vi "ColorReader.vi"(1 "file path (dialog if empty)":path=path "C:/Program Files (x86)/FRC Dashboard", 2 "name or relative path":string="Blue.csv") -> (0 "ColorSettings":T1)   [LabVIEW 2013]
uses:
  <vilib>/Utility/file.llb/Read From Spreadsheet File (string).vi
panel:
  out "LumM":i32
  out "Lum":i32
  out "SatM":i32
  out "Sat":i32
  out "HueM":i32
  out "Hue":i32
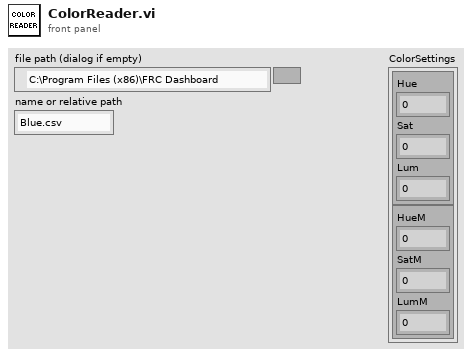
[diagram p1: front panel]
types:
  T1 = cluster{cluster{"Hue":i32, "Sat":i32, "Lum":i32}, cluster{"HueM":i32, "SatM":i32, "LumM":i32}}
  T2 = cluster{"all rows[0]":string, "all rows[1]":string, "all rows[2]":string, "all rows[3]":string, "all rows[4]":string, "all rows[5]":string, "all rows[6]":string, "all rows[7]":string, "all rows[8]":string}
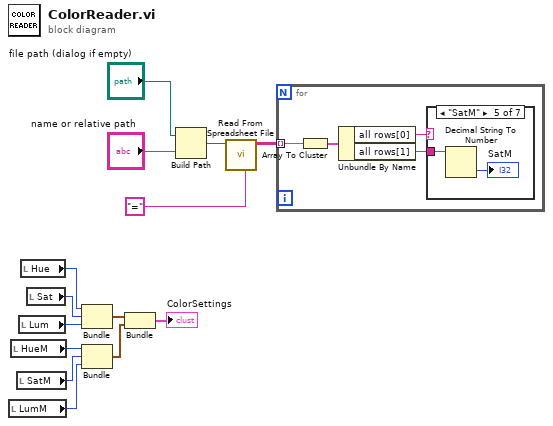
[diagram p0: block diagram]
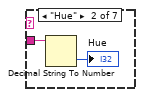
[diagram p3: hidden frame]
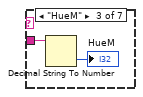
[diagram p4: hidden frame]
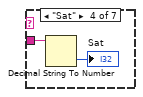
[diagram p5: hidden frame]
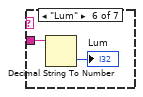
[diagram p6: hidden frame]
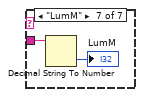
[diagram p7: hidden frame]
diagram:
  n1 = local read "LumM"() -> (w6:i32)
  n2 = local read "HueM"() -> (w9:i32)
  n3 = local read "SatM"() -> (w7:i32)
  n4 = local read "Lum"() -> (w5:i32)
  n5 = local read "Hue"() -> (w8:i32)
  n6 = local read "Sat"() -> (w4:i32)
  n7 = Bundle("Hue"=w8, "Sat"=w4, "Lum"=w5) -> (w10:cluster{"Hue":i32, "Sat":i32, "Lum":i32})  [unwired: 1 in]
  n8 = Bundle("HueM"=w9, "SatM"=w7, "LumM"=w6) -> (w11:cluster{"HueM":i32, "SatM":i32, "LumM":i32})  [unwired: 1 in]
  n9 = Bundle(w10, w11) -> (→"ColorSettings":T1)  [unwired: 1 in]
  n10 = Build Path(base path="file path (dialog if empty)", name or relative path="name or relative path") -> (appended path=w1:path)
  n11 = call-poly <vilib>:"Read From Spreadsheet File.vi"("delimiter (\\t)"="=", "file path (dialog if empty)"=w1) -> ("all rows"=w2:string[][])  [unwired: 5 in, 4 out]
  n12 = for {
    tunnel: w2 -> [w18] mode=indexing
    n13 = Array To Cluster(array=w18) -> (cluster=w17:T2)
    n14 = Unbundle By Name(w17) -> ("all rows[0]"=w16:string, "all rows[1]"=w15:string)
    n15 = case shown="\"SatM\"" w16 {
      tunnel: w15 -> [_ w20 w22 w24 w26 w28 w30]
      frame "", Default {
      }
      frame "Hue" {
        n16 = Decimal String To Number(string=w20) -> (number=→"Hue":i32)  [unwired: 2 in, 1 out]
      }
      frame "HueM" {
        n17 = Decimal String To Number(string=w22) -> (number=→"HueM":i32)  [unwired: 2 in, 1 out]
      }
      frame "Sat" {
        n18 = Decimal String To Number(string=w24) -> (number=→"Sat":i32)  [unwired: 2 in, 1 out]
      }
      frame "SatM" {
        n19 = Decimal String To Number(string=w26) -> (number=→"SatM":i32)  [unwired: 2 in, 1 out]
      }
      frame "Lum" {
        n20 = Decimal String To Number(string=w28) -> (number=→"Lum":i32)  [unwired: 2 in, 1 out]
      }
      frame "LumM" {
        n21 = Decimal String To Number(string=w30) -> (number=→"LumM":i32)  [unwired: 2 in, 1 out]
      }
    }
  }
